vi "camera_state_machine.vi"() -> ()   [LabVIEW 2013]
uses:
  Control 3.ctl
  <userlib>/atmcd32d.llb/AcquisitionMode_mode typedef.ctl
  <userlib>/atmcd32d.llb/ReadMode_mode typedef.ctl
  <userlib>/atmcd32d.llb/TriggerMode_mode typedef.ctl
  System Files/user.lib/atmcd32d.llb/Error Code Enum typedef.ctl
panel:
  out "ImageData":i32[][](array[numeric])
  out "VS Speed Index":i32
  out "Current State":T1
  in  "Tab Control":T2(tab)
  out "Initialize Error Code":u32
  out "Shutdown Error Code":u32
  out "GetDetector Error Code":u32
  out "GetNumberVSSpeeds Error Code":u32
  out "GetVSSpeed Error Code":u32
  out "GetTempRange Error Code":u32
  out "CoolerON Error Code":u32
  out "GetTemperature Error Code":u32
  out "SetAcqMode Error Code":u32
  out "SetReadMode Error Code":u32
  out "Set Exposure Time Error Code":u32
  out "SetVSSpeed Error Code":u32
  out "SetTriggerMode Error Code":u32
  out "SetAccumTimeError":u32
  out "Set#Accum Error":u32
  out "Set#Kinetics Error":u32
  out "SetKineticCycleTime Error":u32
  out "StartAquisition Error Code":u32
  out "GetAcqTimings Error Code":u32
  out "SetImage Error":u32
  out "Get Acq'd Data Error":u32
  out "SetFT Mode Error":u32
  out "Temp Stable":bool
  out "ypixels":i32
  out "xpixels":i32
  out "PCB":u32
  out "Flex":u32
  out "# Vs Speeds":i32
  out "VS Speed (us)":sgl format="%.2f"
  out "maxTemp":i32
  out "minTemp":i32
  out "temperature":i32
  in  "Frame transfer.... ACTIVATE":bool
  in  "Continuous Scanning":bool
  in  "Start Scan":bool
  in  "Acquisition Mode":T3=enum."Single Scan"
  in  "Readout Mode":T4
  in  "Exposure Time (s)":sgl min=0 format="%.2e"
  in  "Trigger Mode":T5
  in  "Accumulation Number":i32=1 min=1 step=1
  in  "Accumulation Cycle Time (s)":sgl format="%.2f"
  in  "Number of Kinetics":i32=1 min=1 step=1
  in  "Kinetic Cycle Time (s)":sgl format="%.2f"
  out "Real Exposure Time (s)":sgl format="%.2f"
  out "Real Kinetic Time (s)":sgl format="%.2f"
  out "Real Accumulate Time (s)":sgl format="%.2f"
  out "Image":i32[][](graph)
  out "Acquisition Status":T6
  out "Get # New Images First":u32
  out "Get # New Images Last":i32
  out "Get # Img Available First":i32
  out "Get # Img Avail. Last":i32
  out "Get Tot Num Img Acq":i32
  in  "Shutdown":bool
  out "error out":errorcluster
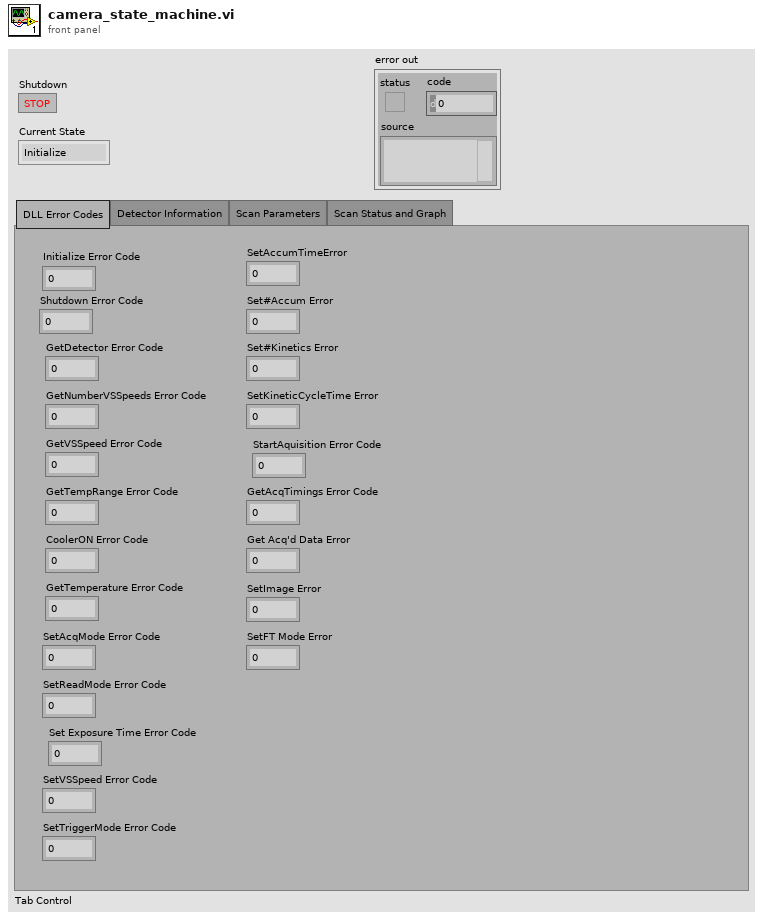
[diagram p1: front panel]
types:
  T1 = typedef "Control 3.ctl" = enum16{"Initialize", "Initialize2", "Switch ON cooler", "Monitor Temperature Drop", "Do Nothing", "Set Acq. Params", "Start Data Acquisition", "Acquiring?", "Get Data", "Shutdown", "Error"}
  T2 = enum32{"DLL Error Codes", "Detector Information", "Scan Parameters", "Scan Status and Graph"}
  T3 = typedef "AcquisitionMode_mode typedef.ctl" = enum16{"Reserved (0)", "Single Scan", "Accumulate", "Kinetics", "Fast Kinetics", "Run Till Abort", "Reserved (6)", "Reserved (7)", "Reserved (8)", "Time Delayed Integration"}
  T4 = typedef "ReadMode_mode typedef.ctl" = enum16{"Full Vertical Binning", "Multi-Track", "Random-Track", "Single-Track", "Image"}
  T5 = typedef "TriggerMode_mode typedef.ctl" = enum16{"Internal", "External", "N/A (2)", "N/A (3)", "N/A (4)", "N/A (5)", "External Start", "External Exposure (Bulb)", "N/A (8)", "External FVB EM", "Software", "N/A (11)", "External Charge Shifting"}
  T6 = typedef "Error Code Enum typedef.ctl" = enum32{"N/A (0)", "DRV_ERROR_CODES", "DRV_SUCCESS", "DRV_VXDNOTINSTALLED", "DRV_ERROR_SCAN", "DRV_ERROR_CHECK_SUM", "DRV_ERROR_FILELOAD", "DRV_UNKNOWN_FUNC", "DRV_ERROR_VXD_INIT", "DRV_ERROR_ADDRESS", "DRV_ERROR_PAGELOCK", "DRV_ERROR_PAGEUNLOCK", "DRV_ERROR_BOARDTEST", "DRV_ERROR_ACK", "DRV_ERROR_UP_FIFO", "DRV_ERROR_PATTERN", "N/A (16)", "DRV_ACQUISITION_ERRORS", "DRV_ACQ_BUFFER", "DRV_ACQ_DOWNFIFO_FULL", "DRV_PROC_UNKONWN_INSTRUCTION", "DRV_ILLEGAL_OP_CODE", "DRV_KINETIC_TIME_NOT_MET", "DRV_ACCUM_TIME_NOT_MET", "DRV_NO_NEW_DATA", "N/A (25)", "DRV_SPOOLERROR", "N/A (27)", "N/A (28)", "N/A (29)", "N/A (30)", "N/A (31)", "N/A (32)", "DRV_TEMPERATURE_CODES", "DRV_TEMPERATURE_OFF", "DRV_TEMPERATURE_NOT_STABILIZED", "DRV_TEMPERATURE_STABILIZED", "DRV_TEMPERATURE_NOT_REACHED", "DRV_TEMPERATURE_OUT_RANGE", "DRV_TEMPERATURE_NOT_SUPPORTED", "DRV_TEMPERATURE_DRIFT", "N/A (41)", "N/A (42)", "N/A (43)", "N/A (44)", "N/A (45)", "N/A (46)", "N/A (47)", "N/A (48)", "DRV_GENERAL_ERRORS", "DRV_INVALID_AUX", "DRV_COF_NOTLOADED", "DRV_FPGAPROG", "DRV_FLEXERROR", "DRV_GPIBERROR", "N/A (55)", "N/A (56)", "N/A (57)", "N/A (58)", "N/A (59)", "N/A (60)", "N/A (61)", "N/A (62)", "N/A (63)", "DRV_DATATYPE", "DRV_DRIVER_ERRORS", "DRV_P1INVALID", "DRV_P2INVALID", "DRV_P3INVALID", "DRV_P4INVALID", "DRV_INIERROR", "DRV_COFERROR", "DRV_ACQUIRING", "DRV_IDLE", "DRV_TEMPCYCLE", "DRV_NOT_INITIALIZED", "DRV_P5INVALID", "DRV_P6INVALID", "DRV_INVALID_MODE", "DRV_INVALID_FILTER", "DRV_I2CERRORS", "DRV_I2CDEVNOTFOUND", "DRV_I2CTIMEOUT", "DRV_P7INVALID", "N/A (84)", "N/A (85)", "N/A (86)", "N/A (87)", "N/A (88)", "N/A (89)", "DRV_IOCERROR", "DRV_VRMVERSIONERROR"}
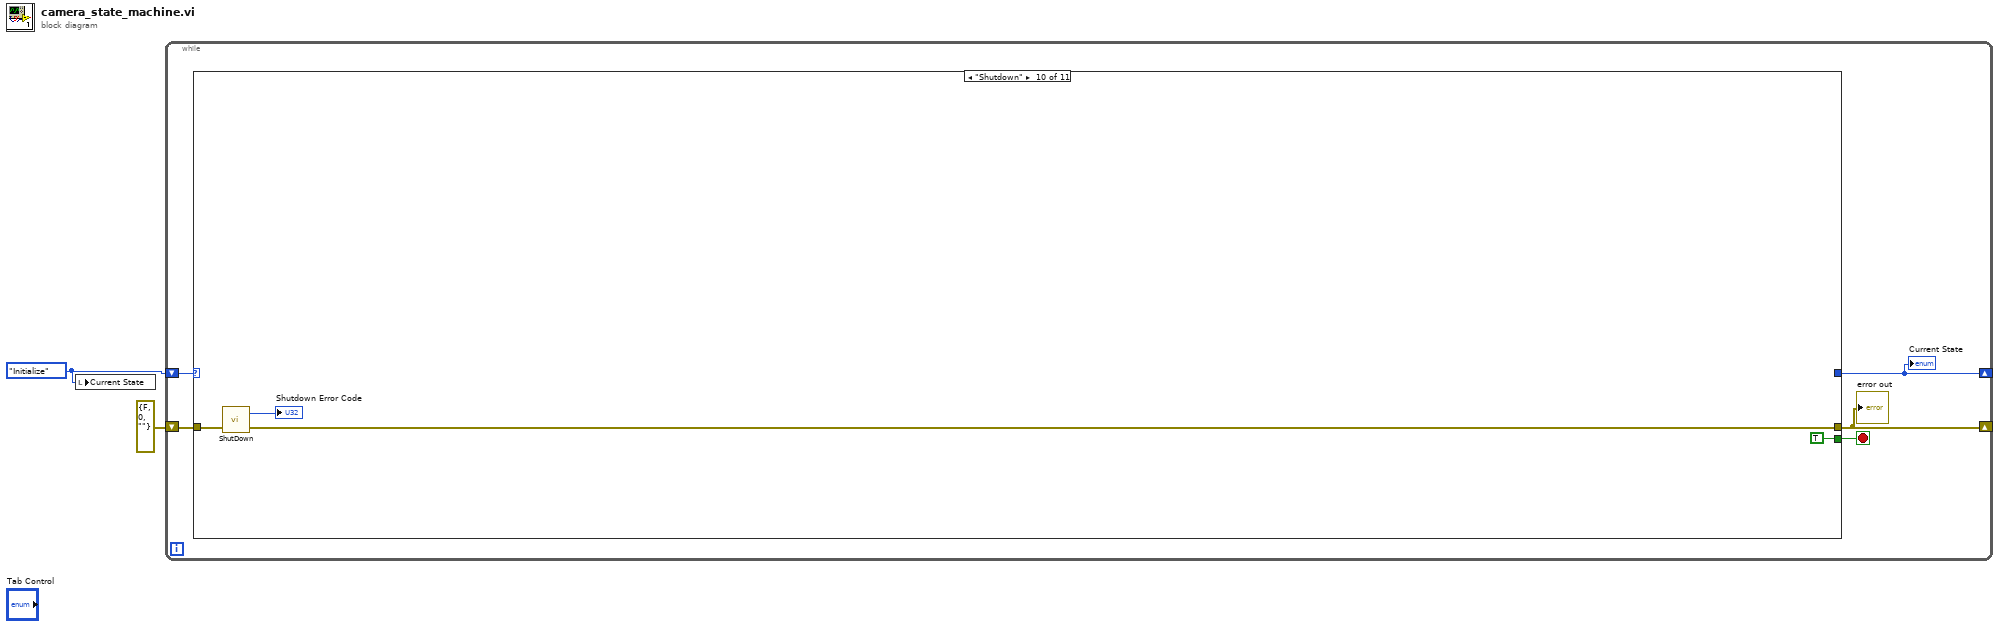
[diagram p0: block diagram]
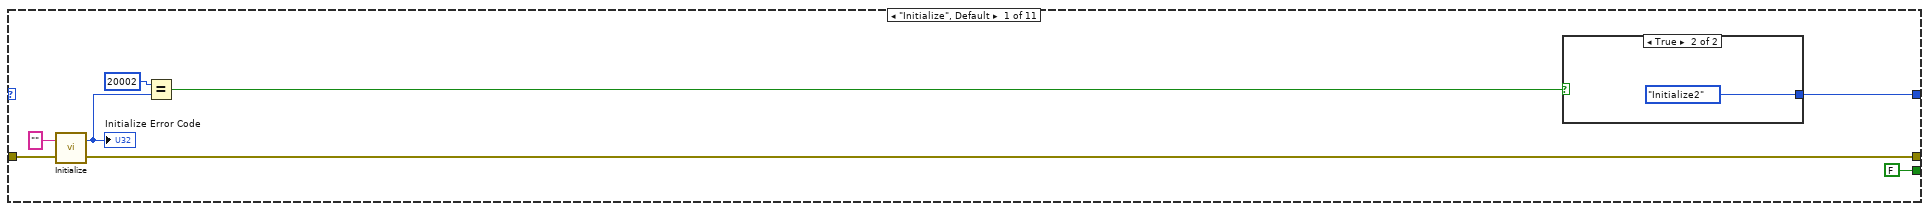
[diagram p2: hidden frame]
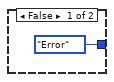
[diagram p3: hidden frame]
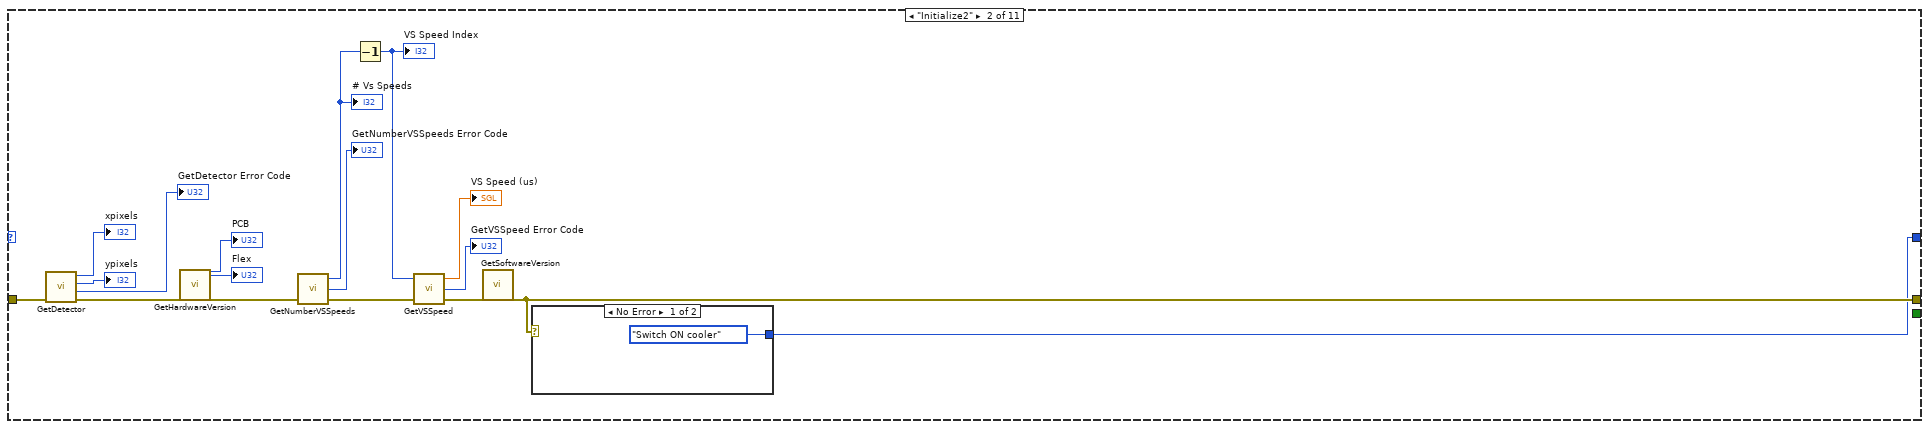
[diagram p4: hidden frame]
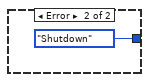
[diagram p5: hidden frame]
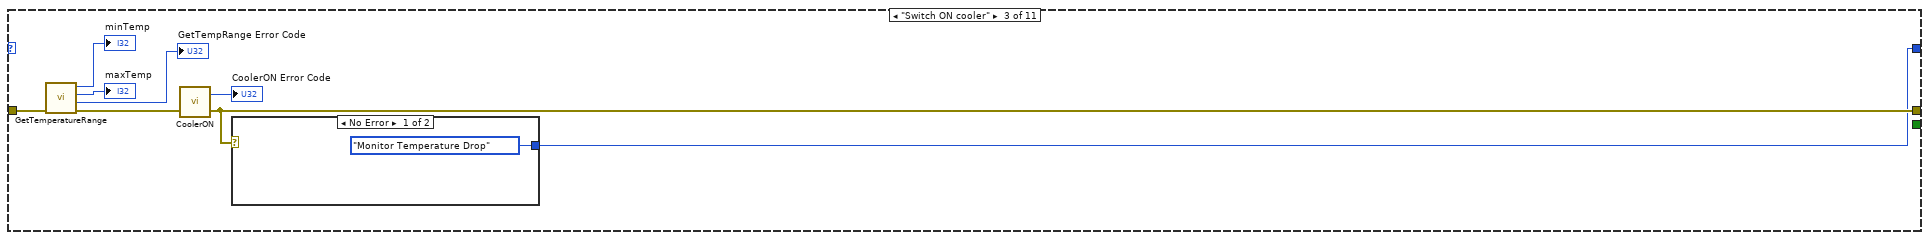
[diagram p6: hidden frame]
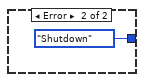
[diagram p7: hidden frame]
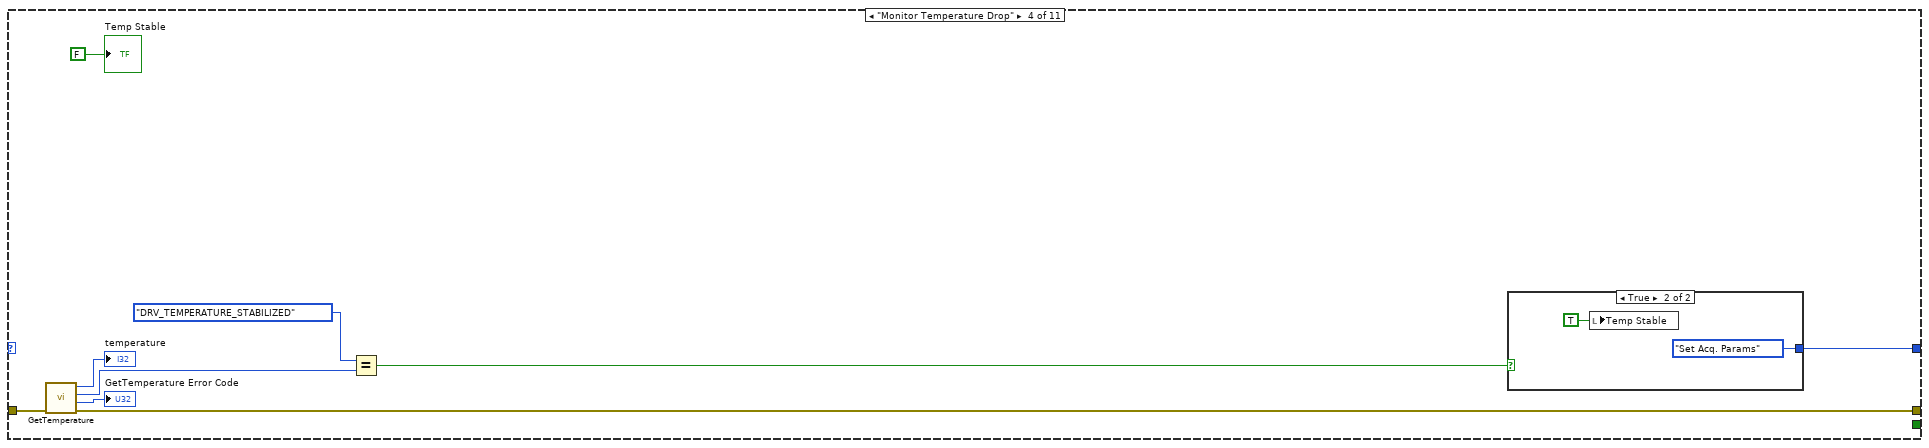
[diagram p8: hidden frame]
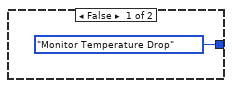
[diagram p9: hidden frame]
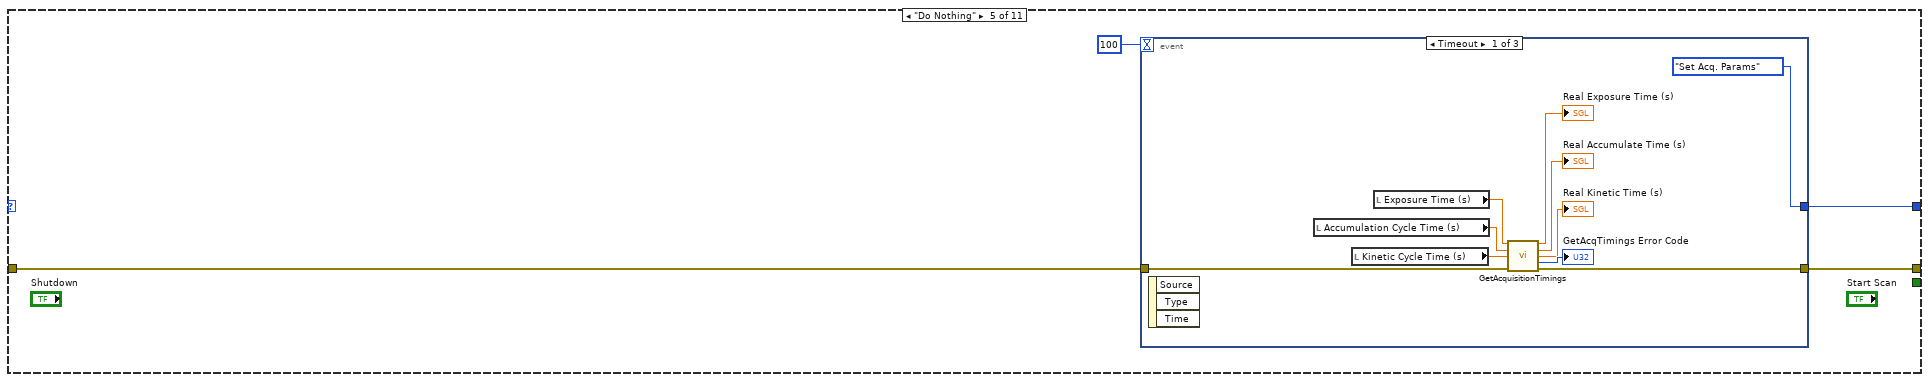
[diagram p10: hidden frame]
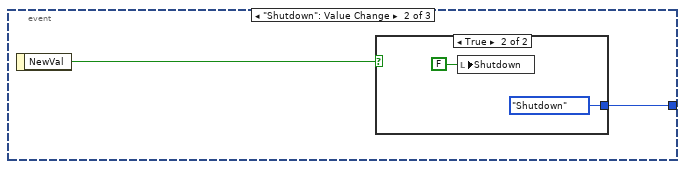
[diagram p11: hidden frame]
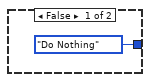
[diagram p12: hidden frame]
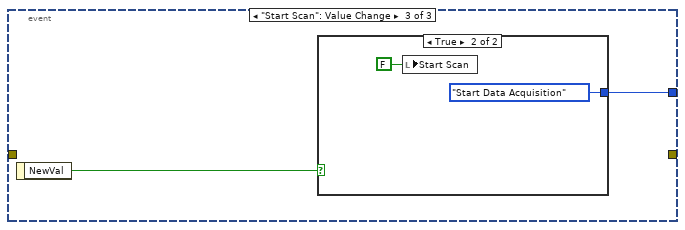
[diagram p13: hidden frame]
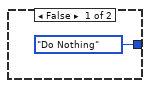
[diagram p14: hidden frame]
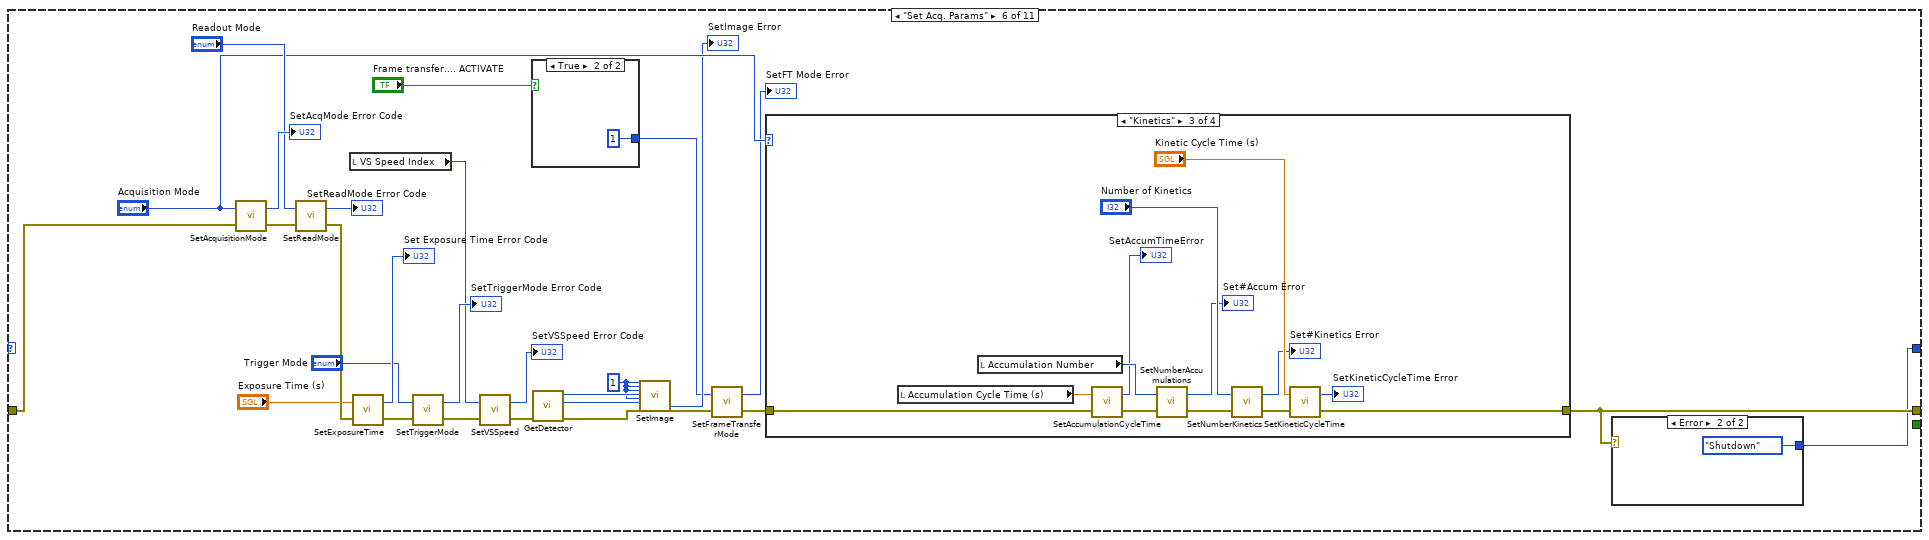
[diagram p15: hidden frame]
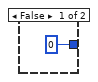
[diagram p16: hidden frame]
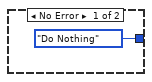
[diagram p17: hidden frame]
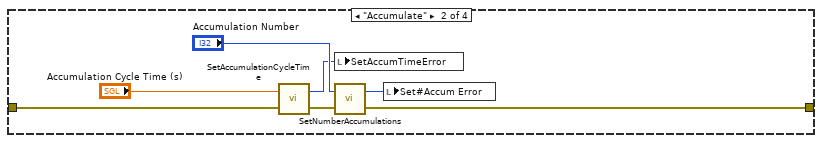
[diagram p19: hidden frame]
diagram:
  w1 = Control_3."Initialize"
  n1 = local write "Current State"(w1) -> ()
  n2 = while {
    shift-right: [w6] -> _
    shift-left: w1 -> [w3]
    shift-right: [w4] -> _
    shift-left: errorcluster {"status"=FALSE, "code"=0, "source"=""} ("error out") -> [w7]
    stop <- w5 stop-if-true
    n3 = case shown="\"Shutdown\"" w3 {
      tunnel: [w14 w19 w38 w54 w60 w95 w138 w147 w173 w203 _] -> w4
      tunnel: w7 -> [w13 w34 w44 w55 w61 w110 w141 w151 w175 w204 _]
      tunnel: [w9 w18 w37 w52 w62 w94 Control_3."Get Data" w148 w176 _ Control_3."Shutdown"] -> w6
      tunnel: [FALSE _ _ _ _ _ _ _ _ TRUE _] -> w5
      frame "Initialize", Default {
        n4 = call <userlib>:"Initialize.vi"("error in (no error)"=w13, "directory (\"\")"="" ("directory (\"\")")) -> ("error out"=w14:errorcluster, "DLL error code"=w12:u32)
        "Initialize Error Code" <- w12
        n5 = Equal?(x=u32 20002, y=w12) -> (x = y?=w10:bool)
        n6 = case shown="True" w10 {
          tunnel: [Control_3."Error" Control_3."Initialize2"] -> w9
          frame False {
          }
          frame True {
          }
        }
      }
      frame "Initialize2" {
        n7 = call <userlib>:"GetDetector.vi"("error in (no error)"=w34) -> ("error out"=w30:errorcluster, "DLL error code"=→"GetDetector Error Code":u32, "ypixels"=→"ypixels":i32, "xpixels"=→"xpixels":i32)  [unwired: 3 in]
        n8 = call <userlib>:"GetHardwareVersion.vi"("error in (no error)"=w30) -> ("PCB"=→"PCB":u32, "Flex"=→"Flex":u32, "error out"=w27:errorcluster)  [unwired: 19 in, 5 out]
        n9 = call <userlib>:"GetNumberVSSpeeds.vi"("error in (no error)"=w27) -> ("error out"=w25:errorcluster, "DLL error code"=→"GetNumberVSSpeeds Error Code":u32, "number"=w23:i32)  [unwired: 2 in]
        "# Vs Speeds" <- w23
        n10 = Decrement(x=w23) -> (x-1=w22:i32)
        "VS Speed Index" <- w22
        n11 = call <userlib>:"GetVSSpeed.vi"("error in (no error)"=w25, "index"=w22) -> ("error out"=w20:errorcluster, "DLL error code"=→"GetVSSpeed Error Code":u32, "speed"=→"VS Speed (us)":sgl)  [unwired: 1 in]
        n12 = call <userlib>:"GetSoftwareVersion.vi"("error in (no error)"=w20) -> ("error out"=w19:errorcluster)  [unwired: 19 in, 7 out]
        n13 = case shown="No Error" w19 {
          tunnel: [Control_3."Switch ON cooler" Control_3."Shutdown"] -> w18
          frame No Error {
          }
          frame Error {
          }
        }
      }
      frame "Switch ON cooler" {
        n14 = call <userlib>:"GetTemperatureRange.vi"("error in (no error)"=w44) -> ("error out"=w40:errorcluster, "DLL error code"=→"GetTempRange Error Code":u32, "maxTemp"=→"maxTemp":i32, "minTemp"=→"minTemp":i32)  [unwired: 3 in]
        n15 = call <userlib>:"CoolerON.vi"("error in (no error)"=w40) -> ("error out"=w38:errorcluster, "DLL error code"=→"CoolerON Error Code":u32)  [unwired: 1 in]
        n16 = case shown="No Error" w38 {
          tunnel: [Control_3."Monitor Temperature Drop" Control_3."Shutdown"] -> w37
          frame No Error {
          }
          frame Error {
          }
        }
      }
      frame "Monitor Temperature Drop" {
        n17 = call <userlib>:"GetTemperature.vi"("error in (no error)"=w55) -> ("error out"=w54:errorcluster, "DLL error code"=→"GetTemperature Error Code":u32, "status"=w51:T6, "temperature"=→"temperature":i32)  [unwired: 3 in]
        n18 = Equal?(x=Error_Code_Enum_typedef."DRV_TEMPERATURE_STABILIZED", y=w51) -> (x = y?=w47:bool)
        n19 = case shown="True" w47 {
          tunnel: [Control_3."Monitor Temperature Drop" Control_3."Set Acq. Params"] -> w52
          frame False {
          }
          frame True {
            n20 = local write "Temp Stable"(TRUE) -> ()
          }
        }
        "Temp Stable" <- FALSE
      }
      frame "Do Nothing" {
        n21 = event shown="[0] Timeout" {
          selector: _ -> [_ _ _]
          dyn-events: _ -> [_ _ _]
          timeout: 100 -> [_ _ _]
          tunnel: [Control_3."Set Acq. Params" w73 w78] -> w62
          tunnel: w61 -> [w64 _ _]
          tunnel: [w63 _ _] -> w60
          event Timeout {
            n22 = event-data() -> ()  [unwired: 1 in, 3 out]
            n23 = local read "Accumulation Cycle Time (s)"() -> (w66:sgl)
            n24 = local read "Kinetic Cycle Time (s)"() -> (w67:sgl)
            n25 = local read "Exposure Time (s)"() -> (w65:sgl)
            n26 = call <userlib>:"GetAcquisitionTimings.vi"("exposure input"=w65, "accumulate input"=w66, "kinetic input"=w67, "error in (no error)"=w64) -> ("exposure"=→"Real Exposure Time (s)":sgl, "accumulate"=→"Real Accumulate Time (s)":sgl, "kinetic"=→"Real Kinetic Time (s)":sgl, "DLL error code"=→"GetAcqTimings Error Code":u32, "error out"=w63:errorcluster)  [unwired: 7 in]
          }
          event "Shutdown": Value Change {
            n27 = event-data() -> ("NewVal"=w74:bool)  [unwired: 1 in]
            n28 = case shown="True" w74 {
              tunnel: [Control_3."Do Nothing" Control_3."Shutdown"] -> w73
              frame False {
              }
              frame True {
                n29 = local write "Shutdown"(FALSE ("Shutdown")) -> ()
              }
            }
          }
          event "Start Scan": Value Change {
            n30 = event-data() -> ("NewVal"=w79:bool)  [unwired: 1 in]
            n31 = case shown="True" w79 {
              tunnel: [Control_3."Do Nothing" Control_3."Start Data Acquisition"] -> w78
              frame False {
              }
              frame True {
                n32 = local write "Start Scan"(FALSE ("Start Scan")) -> ()
              }
            }
          }
        }
      }
      frame "Set Acq. Params" {
        w90 = 1
        n33 = call <userlib>:"SetAcquisitionMode.vi"("error in (no error)"=w110, "mode"="Acquisition Mode") -> ("error out"=w108:errorcluster, "DLL error code"=→"SetAcqMode Error Code":u32)
        n34 = call <userlib>:"SetReadMode.vi"("error in (no error)"=w108, "mode"="Readout Mode") -> ("error out"=w105:errorcluster, "DLL error code"=→"SetReadMode Error Code":u32)
        n35 = local read "VS Speed Index"() -> (w97:i32)
        n36 = call <userlib>:"SetExposureTime.vi"("error in (no error)"=w105, "time"="Exposure Time (s)") -> ("error out"=w102:errorcluster, "DLL error code"=→"Set Exposure Time Error Code":u32)
        n37 = call <userlib>:"SetTriggerMode.vi"("error in (no error)"=w102, "mode"="Trigger Mode") -> ("error out"=w98:errorcluster, "DLL error code"=→"SetTriggerMode Error Code":u32)
        n38 = call <userlib>:"SetVSSpeed.vi"("error in (no error)"=w98, "index"=w97) -> ("error out"=w93:errorcluster, "DLL error code"=→"SetVSSpeed Error Code":u32)
        n39 = case shown="True" "Frame transfer.... ACTIVATE" {
          tunnel: [0 1] -> w86
          frame False {
          }
          frame True {
          }
        }
        n40 = call <userlib>:"GetDetector.vi"("error in (no error)"=w93) -> ("error out"=w92:errorcluster, "ypixels"=w89:i32, "xpixels"=w91:i32)  [unwired: 3 in, 1 out]
        n41 = call "SetImage.vi"("hbin"=w90, "vbin"=w90, "hstart"=w90, "hend"=w91, "vstart"=w90, "vend"=w89, "error in (no error)"=w92) -> ("DLL error code"=→"SetImage Error":u32, "error out"=w85:errorcluster)  [unwired: 19 in]
        n42 = call <userlib>:"SetFrameTransferMode.vi"("error in (no error)"=w85, "mode"=w86) -> ("error out"=w84:errorcluster, "DLL error code"=→"SetFT Mode Error":u32)
        n43 = case shown="\"Kinetics\"" "Acquisition Mode" {
          tunnel: w84 -> [w115 w122 w133 w136]
          tunnel: [w115 w118 w123 w136] -> w95
          frame "Single Scan", Default {
          }
          frame "Accumulate" {
            n44 = call <userlib>:"SetAccumulationCycleTime.vi"("error in (no error)"=w122, "time"="Accumulation Cycle Time (s)") -> ("error out"=w120:errorcluster, "DLL error code"=w117:u32)
            n45 = local write "SetAccumTimeError"(w117) -> ()
            n46 = call <userlib>:"SetNumberAccumulations.vi"("error in (no error)"=w120, "number"="Accumulation Number") -> ("error out"=w118:errorcluster, "DLL error code"=w116:u32)
            n47 = local write "Set#Accum Error"(w116) -> ()
          }
          frame "Kinetics" {
            n48 = local read "Accumulation Cycle Time (s)"() -> (w135:sgl)
            n49 = local read "Accumulation Number"() -> (w134:i32)
            n50 = call <userlib>:"SetAccumulationCycleTime.vi"("error in (no error)"=w133, "time"=w135) -> ("error out"=w132:errorcluster, "DLL error code"=→"SetAccumTimeError":u32)
            n51 = call <userlib>:"SetNumberAccumulations.vi"("error in (no error)"=w132, "number"=w134) -> ("error out"=w131:errorcluster, "DLL error code"=→"Set#Accum Error":u32)
            n52 = call <userlib>:"SetNumberKinetics.vi"("error in (no error)"=w131, "number"="Number of Kinetics") -> ("error out"=w129:errorcluster, "DLL error code"=→"Set#Kinetics Error":u32)
            n53 = call <userlib>:"SetKineticCycleTime.vi"("error in (no error)"=w129, "time"="Kinetic Cycle Time (s)") -> ("error out"=w123:errorcluster, "DLL error code"=→"SetKineticCycleTime Error":u32)
          }
          frame "Run Till Abort" {
          }
        }
        n54 = case shown="Error" w95 {
          tunnel: [Control_3."Do Nothing" Control_3."Shutdown"] -> w94
          frame No Error {
          }
          frame Error {
          }
        }
      }
      frame "Start Data Acquisition" {
        n55 = call <userlib>:"StartAcquisition.vi"("error in (no error)"=w141) -> ("error out"=w139:errorcluster, "DLL error code"=→"StartAquisition Error Code":u32)  [unwired: 1 in]
        n56 = while {
          shift-right: [w145] -> w138
          shift-left: w139 -> [w146]
          stop <- w142 continue-if-true
          n57 = call <userlib>:"GetStatus.vi"("error in (no error)"=w146) -> ("error out"=w145:errorcluster, "status"=w144:T6)  [unwired: 2 in, 1 out]
          "Acquisition Status" <- w144
          n58 = Equal?(x=w144, y=Error_Code_Enum_typedef."DRV_ACQUIRING") -> (x = y?=w142:bool)
        }
      }
      frame "Acquiring?" {
        n59 = flat-sequence {
          tunnel: w151 -> [w162]
          tunnel: [w154] -> w150
          tunnel: w150 -> [w171]
          tunnel: [w163] -> w147
          frame #0 {
            n60 = call <userlib>:"GetNumberNewImages.vi"("error in (no error)"=w162) -> ("error out"=w161:errorcluster, "last"=w158:i32, "first"=w159:u32)  [unwired: 3 in, 1 out]
            n61 = local write "Get # New Images First"(w159) -> ()
            n62 = local write "Get # New Images Last"(w158) -> ()
            n63 = call <userlib>:"GetNumberAvailableImages.vi"("error in (no error)"=w161) -> ("first"=w157:i32, "last"=w156:i32, "error out"=w160:errorcluster)  [unwired: 2 in, 1 out]
            n64 = local write "Get # Img Available First"(w157) -> ()
            n65 = local write "Get # Img Avail. Last"(w156) -> ()
            n66 = call <userlib>:"GetTotalNumberImagesAcquired.vi"("error in (no error)"=w160) -> ("error out"=w154:errorcluster, "index"=w155:i32)  [unwired: 2 in, 1 out]
            n67 = local write "Get Tot Num Img Acq"(w155) -> ()
          }
          frame #1 {
            n68 = local read "ypixels"() -> (w166:i32)
            n69 = local read "xpixels"() -> (w165:i32)
            n70 = local read "ImageData"() -> (w170:i32[][])
            n71 = Multiply(x=w165, y=w166) -> (x*y=w169:i32)
            n72 = Reshape Array(w170, w169) -> (w168:i32[])
            n73 = call <userlib>:"GetMostRecentImage.vi"("error in (no error)"=w171, "size"=w169, "array"=w168) -> ("error out"=w163:errorcluster, "array"=w167:i32[])  [unwired: 1 out]
            n74 = Reshape Array(w167, w166, w165) -> (w164:i32[][])
            n75 = local write "ImageData"(w164) -> ()
            n76 = local write "Image"(w164) -> ()
          }
        }
        n77 = local read "Continuous Scanning"() -> (w149:bool)
        n78 = case shown="True" w149 {
          tunnel: [Control_3."Do Nothing" Control_3."Acquiring?"] -> w148
          frame False {
          }
          frame True {
          }
        }
      }
      frame "Get Data" {
        n79 = flat-sequence {
          tunnel: w175 -> [w180]
          tunnel: [w179] -> w174
          tunnel: w174 -> [w190]
          tunnel: [w189] -> w173
          frame #0 {
            n80 = call <userlib>:"GetNumberNewImages.vi"("error in (no error)"=w180) -> ("error out"=w181:errorcluster, "last"=→"Get # New Images Last":i32, "first"=→"Get # New Images First":u32)  [unwired: 3 in, 1 out]
            n81 = call <userlib>:"GetNumberAvailableImages.vi"("error in (no error)"=w181) -> ("first"=→"Get # Img Available First":i32, "last"=→"Get # Img Avail. Last":i32, "error out"=w182:errorcluster)  [unwired: 2 in, 1 out]
            n82 = call <userlib>:"GetTotalNumberImagesAcquired.vi"("error in (no error)"=w182) -> ("error out"=w179:errorcluster, "index"=→"Get Tot Num Img Acq":i32)  [unwired: 2 in, 1 out]
          }
          frame #1 {
            n83 = local read "Get Tot Num Img Acq"() -> (w195:i32)
            n84 = local read "ypixels"() -> (w200:i32)
            n85 = local read "xpixels"() -> (w194:i32)
            n86 = Multiply(x=w194, y=w200) -> (x*y=w191:i32)
            n87 = Multiply(x=w191, y=w195) -> (x*y=w192:i32)
            n88 = call <userlib>:"GetAcquiredData.vi"("error in (no error)"=w190, "size"=w192) -> ("error out"=w189:errorcluster, "DLL error code"=→"Get Acq'd Data Error":u32, "array"=w196:i32[])  [unwired: 1 in]
            n89 = Multiply(x=w194, y=w195) -> (x*y=w199:i32)
            n90 = Multiply(x=1, y=w196) -> (x*y=w197:i32[])
            n91 = Reshape Array(w197, w200, w199) -> (→"Image" →"ImageData":i32[][])
          }
        }
        n92 = case shown="True" "Continuous Scanning" {
          tunnel: [Control_3."Do Nothing" Control_3."Start Data Acquisition"] -> w176
          frame False {
          }
          frame True {
          }
        }
      }
      frame "Shutdown" {
        n93 = call <userlib>:"ShutDown.vi"("error in (no error)"=w204) -> ("error out"=w203:errorcluster, "DLL error code"=→"Shutdown Error Code":u32)  [unwired: 1 in]
      }
      frame "Error" {
      }
    }
    "error out" <- w4
    "Current State" <- w6
  }
